vi "RichToFlatexternal_driver_wrapper_LogMeasurementResponse.vi"(5 "OutputClusterType":T1, 11 "InputCluster":T2) -> (3 "OutputCluster":T1)   [LabVIEW 2023, in "NIDCPowerSourceDCVoltage_client.lvlib"]
uses:
  external_driver_wrapper_LogMeasurementResponse.ctl
  external_driver_wrapper_LogMeasurementResponse_Flat.ctl
  NIDCPowerSourceDCVoltage_client.lvlib
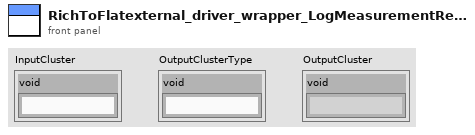
[diagram p1: front panel]
types:
  T1 = typedef "NIDCPowerSourceDCVoltage_client.lvlib/external_driver_wrapper_LogMeasurementResponse_Flat.ctl" = cluster{"void":string}
  T2 = typedef "NIDCPowerSourceDCVoltage_client.lvlib/external_driver_wrapper_LogMeasurementResponse.ctl" = cluster{"void":string}
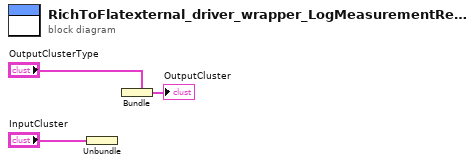
[diagram p0: block diagram]
diagram:
  n1 = Unbundle "Unbundle"("InputCluster") -> ()  [unwired: 1 out]
  n2 = Bundle "Bundle"(cluster="OutputClusterType") -> (→"OutputCluster":T1)  [unwired: 1 in]
